vi "Optimizer.vi"(7 "Mass Flow (lbm/min) vs. Pressure Drop (inH2O) - Real Data":dbl[][](array[numeric])=[[0.5, 0.015], [1.0, 0.062], [1.5, 0.141], [2.0, 0.252], [2.5, 0.395], [3.5, 0.778]], 8 "error in":errorcluster, 10 "Tuners":T1={"Inlet Diameter (in)"=0.0, "Outlet Diameter (in)"=0.0, "Length (in)"=0.0, "Pipe_Diameter (in)"=0.0, "D_h (in)"=0.0, "OAR"=1.0, "Run Optimizer"=FALSE} {"OAR" items=["0.92"=0.92, "0.93"=0.93, "0.94"=0.94, "0.95"=0.95, "0.96"=0.96]; "D_h (in)" items=["0.0625"=0.0625, "0.125"=0.125, "0.250"=0.25]; "Pipe_Diameter (in)" min=0.1 max=6.0 scale=0.0..6.0 scale format="%#_3g"; "Length (in)" min=0.1 max=5.0 scale=0.0..6.0 scale format="%#_3g"; "Outlet Diameter (in)" min=0.1 max=5.0 scale=0.0..5.0 scale format="%#_3g"; "Inlet Diameter (in)" min=0.1 max=5.0 scale=0.0..5.0}, 11 "System Configuration":T2={"P_amb (psia)"=0.125, "T_in (Deg F)"=14.7, "R_air (ft*lbf)/(lbm*R)"=530.0, "g_c (lbm*ft)/(lbf*s^2)"=53.35, "specific heat ratio"=32.17, "Viscousity (lbm)/(ft*s)"=1.4, "Cd"=0.95, "Mass Flow (lbm/min) vs. Pressure Drop (inH2O) - Real Data"=[[0.5, 0.015], [1.0, 0.062], [1.5, 0.141], [2.0, 0.252], [2.5, 0.395], [3.5, 0.778]]} {"Mass Flow (lbm/min) vs. Pressure Drop (inH2O) - Real Data" format="%_3g"; "P_amb (psia)" format="%#_4g"}) -> (0 "error out":errorcluster, 3 "optimized_diameter":dbl)   [LabVIEW 2025]
uses:
  controls/Constants.ctl
  controls/Tuners.ctl
panel:
  # "Honeycomb Parameters"
  # "Orifice Parameters"
  # "Pipe Parameters"
  # "AIRFLOW SIMULATOR"
  # "Mass_flowrate"
  # "Pipe_Diameter"
  # "Outlet_Diameter"
  # "Inlet_Diameter"
  # "Honeycomb_Length"
  # "Empirical Flow Path Data"
  # "Mass Flow\n (lbm/min)"
  # "Pressure Drop \n    (inH2O)"
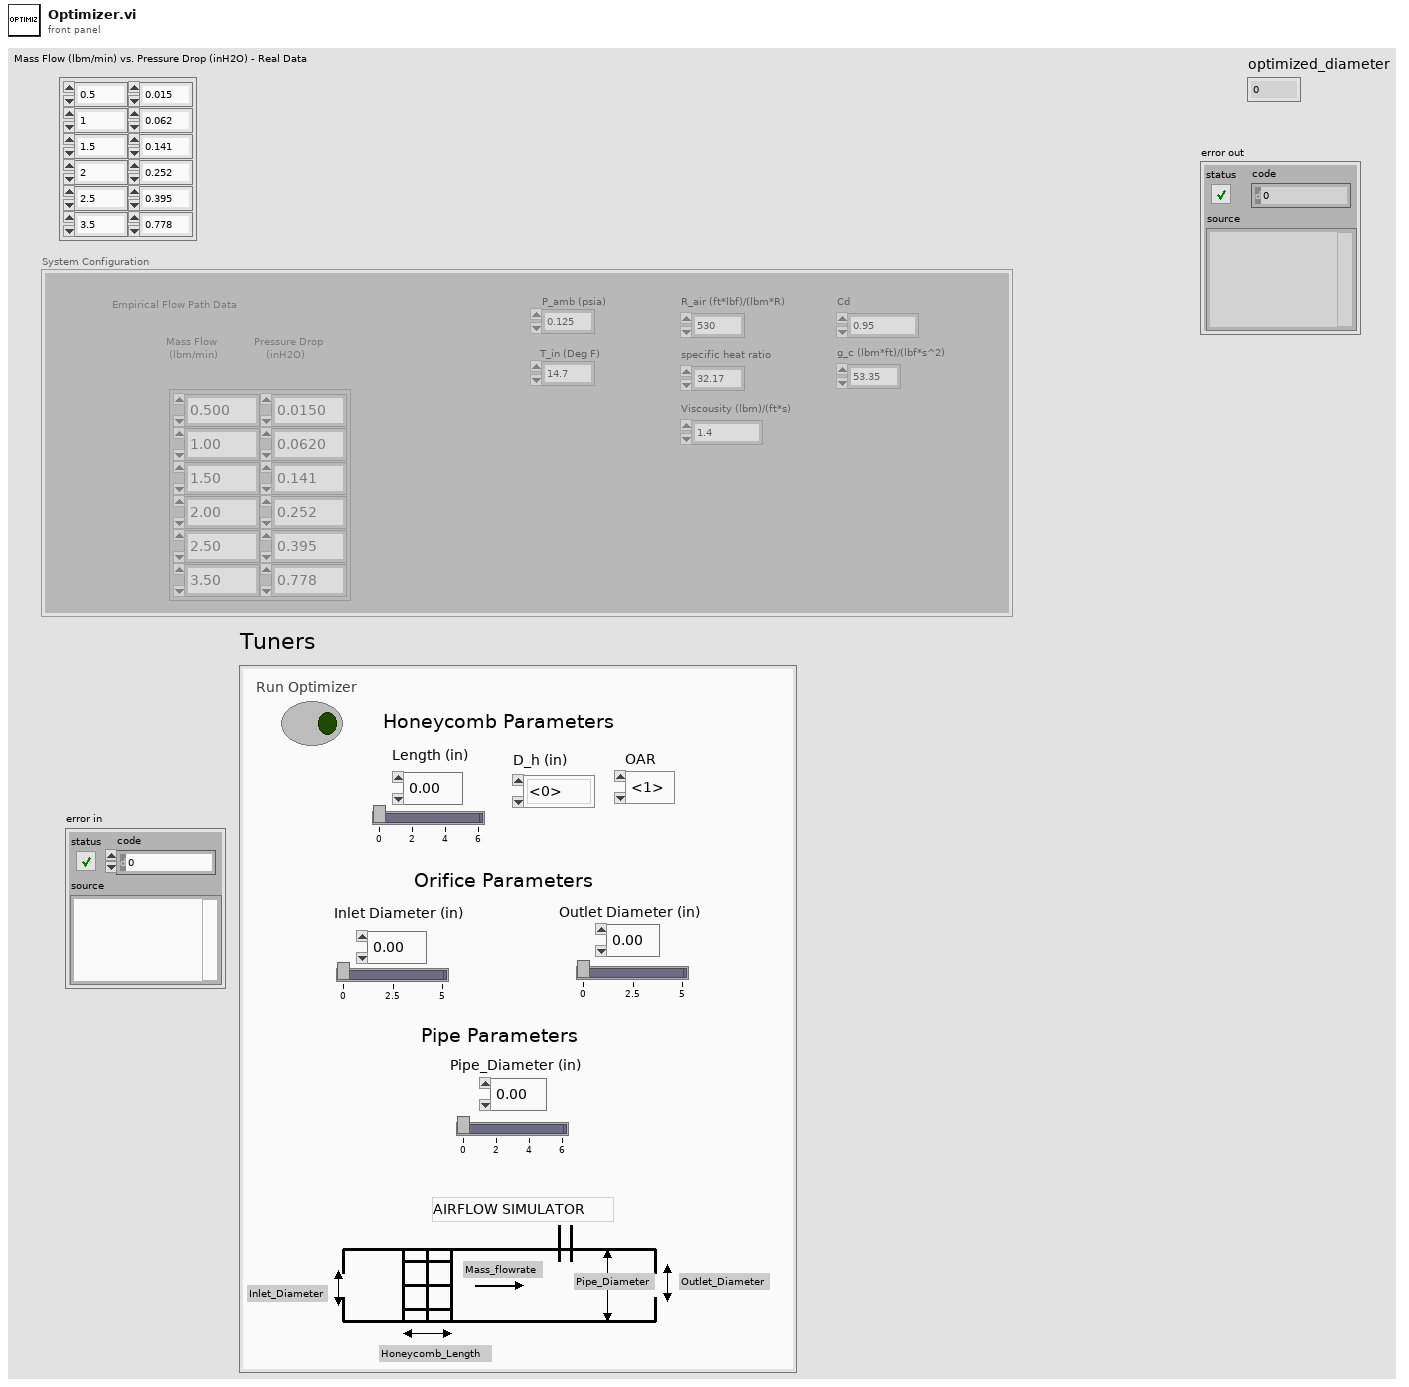
[diagram p1: front panel]
types:
  T1 = typedef "Tuners.ctl" = cluster{"Inlet Diameter (in)":dbl, "Outlet Diameter (in)":dbl, "Length (in)":dbl, "Pipe_Diameter (in)":dbl, "D_h (in)":dbl, "OAR":dbl, "Run Optimizer":bool}
  T2 = typedef "Constants.ctl" = cluster{"P_amb (psia)":dbl, "T_in (Deg F)":dbl, "R_air (ft*lbf)/(lbm*R)":dbl, "g_c (lbm*ft)/(lbf*s^2)":dbl, "specific heat ratio":dbl, "Viscousity (lbm)/(ft*s)":dbl, "Cd":dbl, "Mass Flow (lbm/min) vs. Pressure Drop (inH2O) - Real Data":dbl[][]}
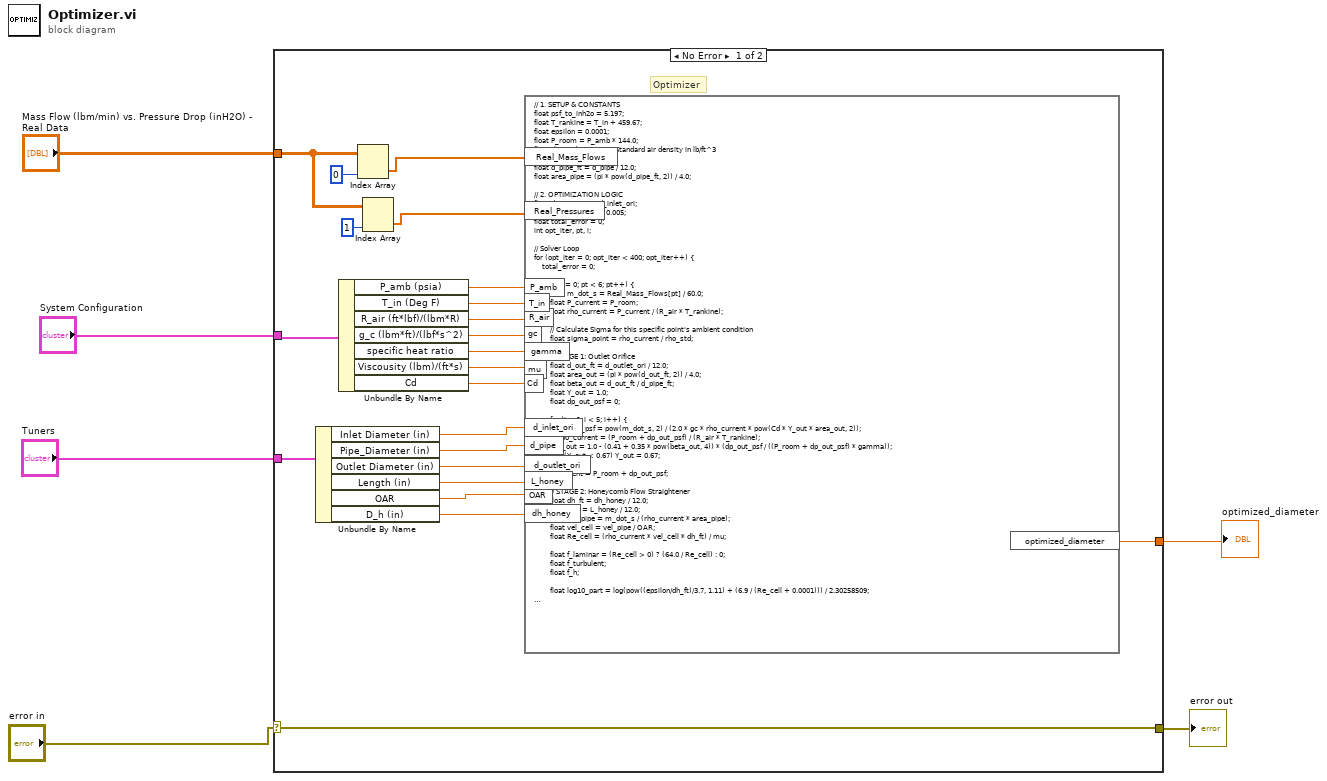
[diagram p0: block diagram]
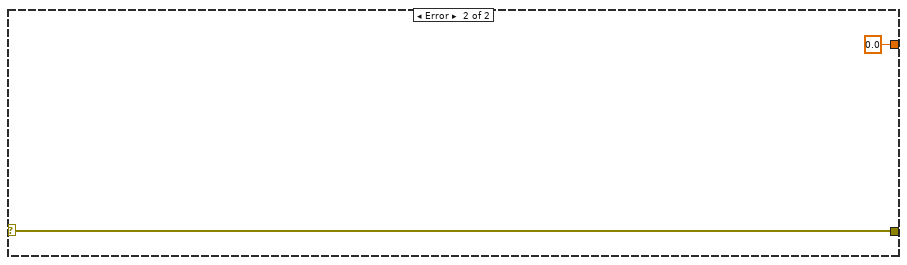
[diagram p2: hidden frame]
diagram:
  n1 = case shown="No Error" "error in" {
    selector: "error in" -> [w9 w30]
    tunnel: "Mass Flow (lbm/min) vs. Pressure Drop (inH2O) - Real Data" -> [w26 _]
    tunnel: [w12 0.0 ("optimized_diameter")] -> w5
    tunnel: "System Configuration" -> [w11 _]
    tunnel: "Tuners" -> [w10 _]
    tunnel: [w9 w30] -> w3
    frame No Error {
      # "Optimizer"
      n2 = Unbundle By Name(w10) -> ("Inlet Diameter (in)"=w16:dbl, "Pipe_Diameter (in)"=w15:dbl, "Outlet Diameter (in)"=w14:dbl, "Length (in)"=w13:dbl, "OAR"=w8:dbl, "D_h (in)"=w7:dbl)
      n3 = Unbundle By Name(w11) -> ("P_amb (psia)"=w23:dbl, "T_in (Deg F)"=w22:dbl, "R_air (ft*lbf)/(lbm*R)"=w21:dbl, "g_c (lbm*ft)/(lbf*s^2)"=w20:dbl, "specific heat ratio"=w19:dbl, "Viscousity (lbm)/(ft*s)"=w18:dbl, "Cd"=w17:dbl)
      n4 = Index Array(array=w26, index (col)=0) -> (element=w25:dbl[])  [unwired: 1 in]
      n5 = Index Array(array=w26, index (col)=1) -> (element=w24:dbl[])  [unwired: 1 in]
      n6 = formula code="// 1. SETUP & CONSTANTS\nfloat psf_to_inh2o = 5.197;\nfloat T_rankine = T_in + 459.67; \nfloat epsilon = 0.0001; \nfloat P_room = P_amb * 144.0; \nfloat rho_std = 0.075; // Standard air density in lb/ft^3\n\nfloat d_pipe_ft = d_pipe / 12.0;\nfloat area_pipe = (pi * pow(d_pipe_ft, 2)) / 4.0;\n\n// 2. OPTIMIZATION LOGIC\nfloat d_in_guess = d_inlet_ori; \nfloat learning_rate = 0.005; \nfloat total_error = 0;\nint opt_iter, pt, i;\n\n// Solver Loop\nfor (opt_iter = 0; opt_iter < 400; opt_iter++) {\n    total_error = 0;\n    \n    for (pt = 0; pt < 6; pt++) {\n        float m_dot_s = Real_Mass_Flows[pt] / 60.0; \n        float P_current = P_room;\n        float rho_current = P_current / (R_air * T_rankine);\n        \n        // Calculate Sigma for this specific point's ambient condition\n        float sigma_point = rho_current / rho_std;\n\n        // STAGE 1: Outlet Orifice\n        float d_out_ft = d_outlet_ori / 12.0;\n        float area_out = (pi * pow(d_out_ft, 2)) / 4.0;\n        float beta_out = d_out_ft / d_pipe_ft;\n        float Y_out = 1.0;\n        float dp_out_psf = 0;\n        \n        for (i = 0; i < 5; i++) {\n            dp_out_psf = pow(m_dot_s, 2) / (2.0 * gc * rho_current * pow(Cd * Y_out * area_out, 2));\n            rho_current = (P_room + dp_out_psf) / (R_air * T_rankine);\n            Y_out = 1.0 - (0.41 + 0.35 * pow(beta_out, 4)) * (dp_out_psf / ((P_room + dp_out_psf) * gamma));\n            if (Y_out < 0.67) Y_out = 0.67;\n        }\n        P_current = P_room + dp_out_psf;\n\n        // STAGE 2: Honeycomb Flow Straightener\n        float dh_ft = dh_honey / 12.0;\n        float L_ft = L_honey / 12.0; \n        float vel_pipe = m_dot_s / (rho_current * area_pipe);\n        float vel_cell = vel_pipe / OAR; \n        float Re_cell = (rho_current * vel_cell * dh_ft) / mu;\n        \n        float f_laminar = (Re_cell > 0) ? (64.0 / Re_cell) : 0;\n        float f_turbulent;\n        float f_h;\n\n        float log10_part = log(pow((epsilon/dh_ft)/3.7, 1.11) + (6.9 / (Re_cell + 0.0001))) / 2.30258509;\n        f_turbulent = pow(1.0 / (-1.8 * log10_part), 2);\n\n        if (Re_cell < 2000) f_h = f_laminar;\n        else if (Re_cell > 3000) f_h = f_turbulent;\n        else f_h = (1.0 - ((Re_cell - 2000) / 1000.0)) * f_laminar + ((Re_cell - 2000) / 1000.0) * f_turbulent;\n\n        P_current += f_h * (L_ft / dh_ft) * (rho_current * pow(vel_cell, 2)) / (2.0 * gc);\n        rho_current = P_current / (R_air * T_rankine);\n\n        // STAGE 3: Inlet Orifice\n        float d_in_ft = d_in_guess / 12.0;\n        float area_in = (pi * pow(d_in_ft, 2)) / 4.0;\n        float beta_in = d_in_ft / d_pipe_ft;\n        float Y_in = 1.0;\n        float dp_in_psf = 0;\n        \n        for (i = 0; i < 5; i++) {\n            dp_in_psf = pow(m_dot_s, 2) / (2.0 * gc * rho_current * pow(Cd * Y_in * area_in, 2));\n            rho_current = (P_current + dp_in_psf) / (R_air * T_rankine);\n            Y_in = 1.0 - (0.41 + 0.35 * pow(beta_in, 4)) * (dp_in_psf / ((P_current + dp_in_psf) * gamma));\n            if (Y_in < 0.67) Y_in = 0.67;\n        }\n        \n        // CONVERT TO SIGMA DELTA PRESSURE\n        // P_final - P_room is the raw delta P. We multiply by sigma to get sigma-dP.\n        float raw_dp_inh2o = (P_current + dp_in_psf - P_room) / psf_to_inh2o;\n        float sigma_dp = raw_dp_inh2o * sigma_point;\n        \n        total_error += (Real_Pressures[pt] - sigma_dp);\n    }\n\n    d_in_guess -= (total_error / 6.0) * learning_rate;\n    if (d_in_guess < 0.1) d_in_guess = 0.1;\n    if (d_in_guess > d_pipe) d_in_guess = d_pipe * 0.95;\n    if (abs(total_error) < 0.005) break; \n}\n\noptimized_diameter = d_in_guess;"("d_inlet_ori"=w16, "d_pipe"=w15, "gamma"=w19, "P_amb"=w23, "OAR"=w8, "mu"=w18, "d_outlet_ori"=w14, "L_honey"=w13, "gc"=w20, "R_air"=w21, "T_in"=w22, "dh_honey"=w7, "Cd"=w17, "Real_Pressures"=w24, "Real_Mass_Flows"=w25) -> ("optimized_diameter"=w12:dbl)
    }
    frame Error {
    }
  }
  "optimized_diameter" <- w5
  "error out" <- w3
